vi "triggerStopServerOcc.vi"(8 "error in (no error)":errorcluster, 11 "TcpServerCmd in":refnum<class "TcpServerCmd.lvclass">) -> (0 "error out":errorcluster, 3 "TcpServerCmd out":refnum<class "TcpServerCmd.lvclass">)   [LabVIEW 2018, in "TcpServerCmd.lvclass"]
doc: "Set the stopServer occurrence to stop the runServer.vi."
uses:
  TcpServerCmd.lvclass
  home/pcortes/github/ts_labview_tcp_json/src/TcpServerBase/TcpServerBase.lvclass
  TcpServerBase/TcpServerBase.lvclass
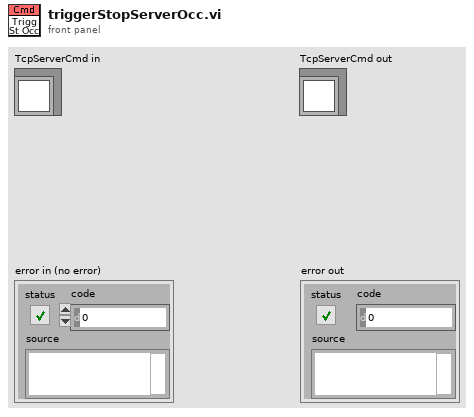
[diagram p1: front panel]
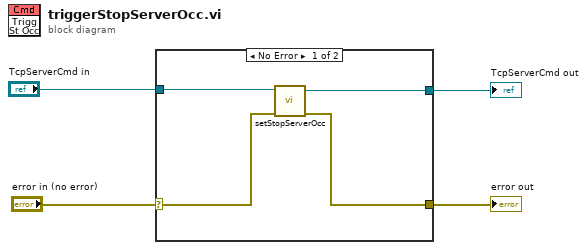
[diagram p0: block diagram]
diagram:
  n1 = case shown="No Error" "error in (no error)" {
    selector: "error in (no error)" -> [w6 w10]
    tunnel: "TcpServerCmd in" -> [w8 w9]
    tunnel: [w5 w10] -> w2
    tunnel: [w7 w9] -> w1
    frame No Error {
      n2 = call "setStopServerOcc.vi"("error in (no error)"=w6, "TcpServerBase in"=w8) -> ("error out"=w5:errorcluster, "TcpServerBase out"=w7:refnum<class "TcpServerCmd.lvclass">)  [unwired: 8 in]
    }
    frame Error {
    }
  }
  "error out" <- w2
  "TcpServerCmd out" <- w1
